vi "DB Monitor.vi"() -> ()   [LabVIEW 2014]
uses:
  <vilib>/drjdpowell/SQLite Library/SQL Statement/SQLITE Datatype.ctl
  <vilib>/drjdpowell/SQLite Library/SQL Statement/SQL Statement.lvclass/SQL Statement.ctl
  <vilib>/drjdpowell/SQLite Library/SQL Connection/Open (string).vi
  <vilib>/drjdpowell/SQLite Library/SQL Statement/Get Column Count.vi
  <vilib>/drjdpowell/SQLite Library/SQL Statement/Get Column Names.vi
  <vilib>/drjdpowell/SQLite Library/SQL Statement/Column Type.vi
  <vilib>/drjdpowell/SQLite Library/SQL Statement/Write Next Column.vi
  <vilib>/drjdpowell/SQLite Library/SQL Statement/Get Column Name.vi
  <vilib>/drjdpowell/SQLite Library/SQL Connection/Execute SQL (No results).vi
  <vilib>/drjdpowell/SQLite Library/SQL Statement/Error Message.vi
  <vilib>/drjdpowell/SQLite Library/SQL Statement/Column String.vi
  <vilib>/drjdpowell/SQLite Library/SQL Connection/Connection.lvclass
  <vilib>/drjdpowell/SQLite Library/SQL Statement/SQL Statement.lvclass
  <vilib>/drjdpowell/SQLite Library/SQLite.lvlib
panel:
  out "Value":string
  out "Current Row":i32
  out "Total Row Count":i32
  out "Data type":T1
  out "LVTime":string
  out "LVTIme type":T1
  out "name":string
  out "name type":T1
  out "pk":string
  out "error out":errorcluster
  in  "stop":bool
  out "Column:Count":i32
  out "Column:Names":string[](array[string])
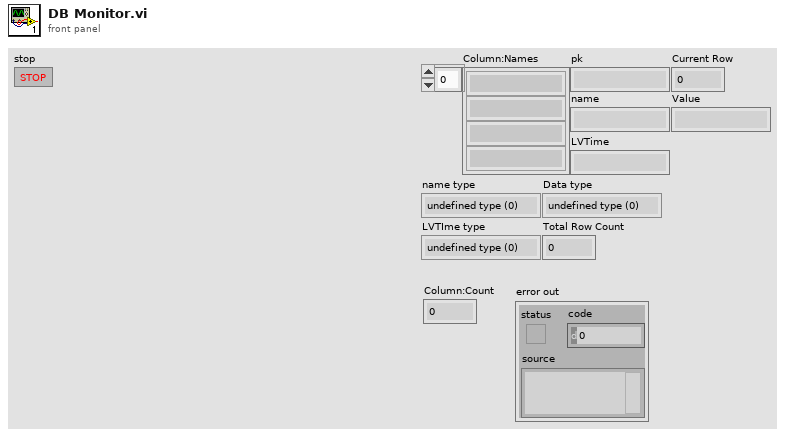
[diagram p1: front panel]
types:
  T1 = typedef "SQLite.lvlib/SQLITE Datatype.ctl" = enum32{"undefined type (0)", "SQLITE_INTEGER", "SQLITE_FLOAT", "SQLITE3_TEXT", "SQLITE_BLOB", "SQLITE_NULL", "undefined type"}
  T2 = enum16{"New or existing", "Existing", "Read only"}
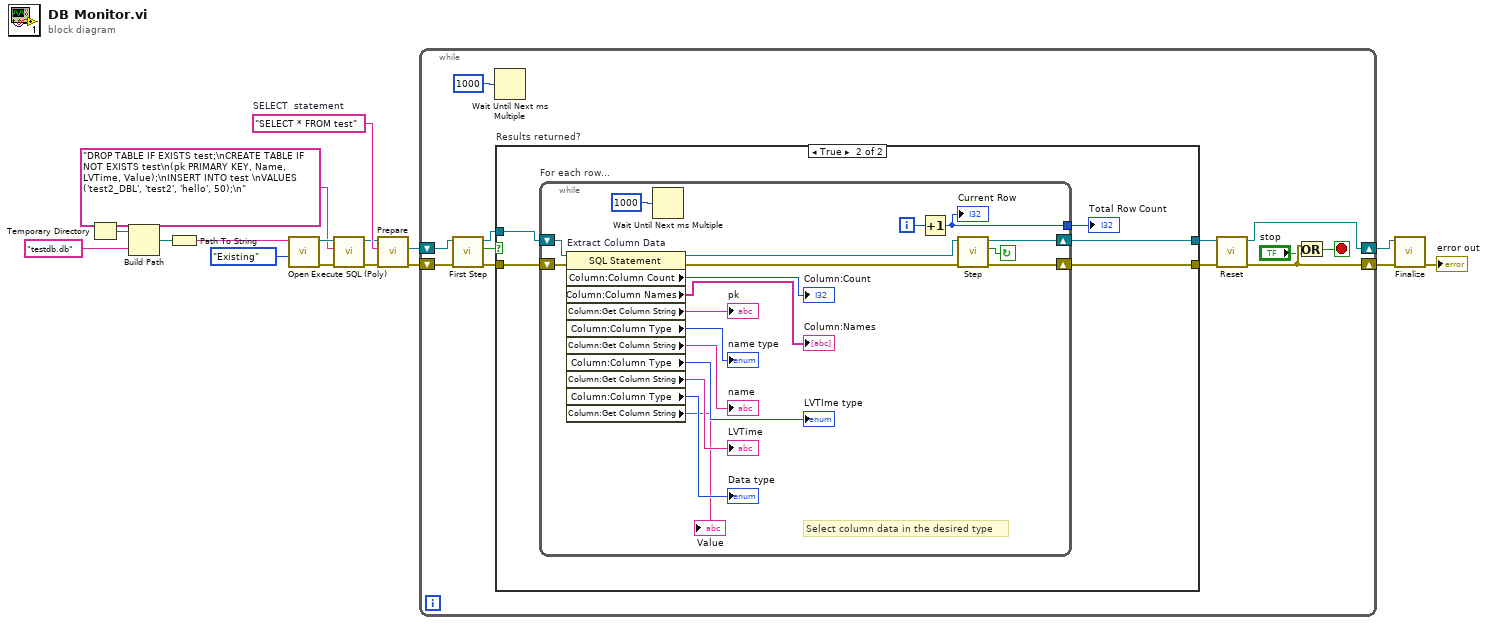
[diagram p0: block diagram]
diagram:
  w12 = "SELECT * FROM test"  # SELECT  statement
  n1 = Temporary Directory() -> (w16:path)
  n2 = Build Path(base path=w16, name or relative path="testdb.db") -> (appended path=w14:path)
  n3 = Path To String(path=w14) -> (string=w13:string)
  n4 = call-poly <vilib>:"Open.vi"("File Option"=T2."Existing", "db file"=w13) -> ("error out"=w4:errorcluster, "SQLite Connection out"=w5:refnum<class "Connection.lvclass">)  [unwired: 8 in]
  n5 = call-poly <vilib>:"Execute SQL (Poly).vi"("error in (no error)"=w4, "SQL"="DROP TABLE IF EXISTS test;\nCREATE TABLE IF NOT EXISTS test\n(pk PRIMARY KEY, Name, LVTime, Value);\nINSERT INTO test \nVALUES ('test2_DBL', 'test2', 'hello', 50);\n", "SQLite Connection in"=w5) -> ("error out"=w3:errorcluster, "SQLite Connection out"=w2:refnum<class "Connection.lvclass">)  [unwired: 7 in]
  n6 = call <vilib>:"Prepare.vi"("error in (no error)"=w3, "SQL"=w12, "SQLite Connection in"=w2) -> ("error out"=w11:errorcluster, "SQL Statement out"=w10:refnum<class "SQL Statement.lvclass">)  [unwired: 4 in, 3 out]
  n7 = while {
    shift-right: [w21] -> w9
    shift-left: w10 -> [w25]
    shift-right: [w19] -> w8
    shift-left: w11 -> [w26]
    stop <- w17 stop-if-true
    n8 = call <vilib>:"First Step.vi"("error in (no error)"=w26, "SQL Statement in"=w25) -> ("error out"=w23:errorcluster, "Row returned"=w22:bool, "SQL Statement out"=w24:refnum<class "SQL Statement.lvclass">)  [unwired: 7 in]
    n9 = Wait Until Next ms Multiple(millisecond multiple=u32 1000) -> ()  [unwired: 1 out]
    n10 = case "Results returned?" shown="True" w22 {
      tunnel: [w30 w35] -> w27
      tunnel: [w29 w34] -> w28
      tunnel: w24 -> [w30 w33]
      tunnel: w23 -> [w29 w32]
      frame False {
      }
      frame True {
        n11 = while "For each row..." {
          shift-right: [w54] -> w35
          shift-left: w33 -> [w51]
          shift-right: [w52] -> w34
          shift-left: w32 -> [w50]
          tunnel: [w37] -> w31
          i -> [w38]
          stop <- w49 continue-if-true
          # "Select column data in the desired type"
          n12 = property on="Extract Column Data" class="SQL Statement"(reference=w51, error in=w50) -> (reference out=w48:refnum<class "SQL Statement.lvclass">, error out=w53:errorcluster, "Column:Column Count"=→"Column:Count":i32, "Column:Column Names"=→"Column:Names":string[], "Column:Get Column String"=→"pk":string, "Column:Column Type"=→"name type":T1, "Column:Get Column String"=→"name":string, "Column:Column Type"=→"LVTIme type":T1, "Column:Get Column String"=→"LVTime":string, "Column:Column Type"=→"Data type":T1, "Column:Get Column String"=→"Value":string)
          n13 = Wait Until Next ms Multiple(millisecond multiple=u32 1000) -> ()  [unwired: 1 out]
          n14 = Increment(x=w38) -> (x+1=w37:i32)
          "Current Row" <- w37
          n15 = call <vilib>:"Step.vi"("error in (no error)"=w53, "SQL Statement in"=w48) -> ("error out"=w52:errorcluster, "Row returned"=w49:bool, "SQL Statement out"=w54:refnum<class "SQL Statement.lvclass">)  [unwired: 7 in]
        }
        "Total Row Count" <- w31
      }
    }
    n16 = call <vilib>:"Reset.vi"("error in (no error)"=w28, "SQL Statement in"=w27) -> ("error out"=w19:errorcluster, "SQL Statement out"=w21:refnum<class "SQL Statement.lvclass">)  [unwired: 8 in]
    n17 = Or(x=w19, y="stop") -> (x .or. y?=w17:bool)
  }
  n18 = call <vilib>:"Finalize.vi"("error in (no error)"=w8, "SQL Statement in"=w9) -> ("error out"=→"error out":errorcluster)  [unwired: 9 in]
